vi "ClearProcessDefault.vi"(8 "error in (no error)":errorcluster) -> (0 "error out":errorcluster)   [LabVIEW 2026, in "Lumberjack.lvlib"]
doc: "Clears the process-default Logger so ResolveLogger returns no instance until the next Initialize. Called by Shutdown during teardown so a stale default does not outlive the manager it referenced. Idempotent: clearing when no default is set is a no-op."
uses:
  Lumberjack.lvlib
  Public/Logger.lvclass/Logger.lvclass
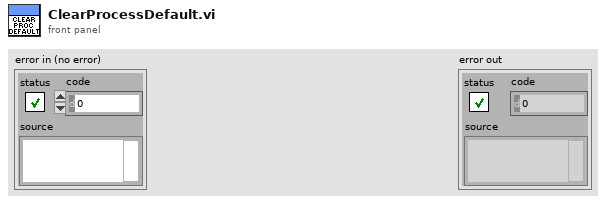
[diagram p1: front panel]
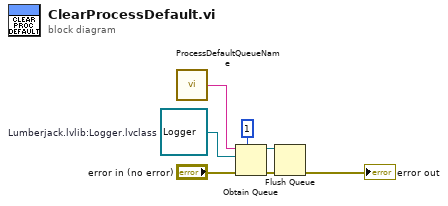
[diagram p0: block diagram]
diagram:
  w2 = refnum<class "Logger.lvclass"> refnum  # Lumberjack.lvlib:Logger.lvclass
  n1 = call "ProcessDefaultQueueName.vi"() -> ("processDefaultQueueName"=w3:string)
  n2 = Obtain Queue(max queue size (-1, unlimited)=1, name (unnamed)=w3, element data type=w2, error in (no error)="error in (no error)") -> (queue out=w4:refnum<queue>, error out=w6:errorcluster)  [unwired: 1 in, 1 out]
  n3 = Flush Queue(queue=w4, error in (no error)=w6) -> (error out=→"error out":errorcluster)  [unwired: 2 out]
